vi "to posint fixint.vi"(8 "error in":errorcluster, 11 "bytes":u8[](array[numeric]) format="%b") -> (0 "error out":errorcluster, 2 "fix int":u8, 3 "remaining bytes":u8[](array[numeric]))   [LabVIEW 2020, in "MessagePack.lvlib" / "MessagePack.lvclass"]
uses:
  MessagePack.lvclass
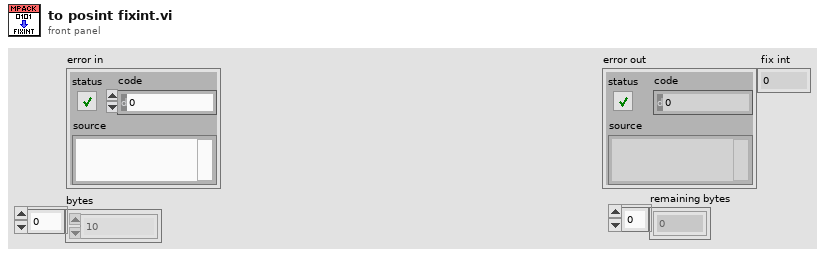
[diagram p1: front panel]
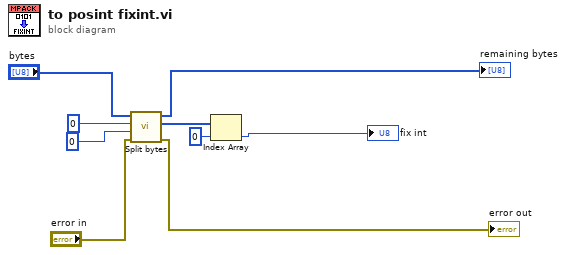
[diagram p0: block diagram]
diagram:
  n1 = call "Split bytes.vi"("error in"="error in", "End index"=0, "Start index"=0, "bytes in"="bytes") -> ("error out"=→"error out":errorcluster, "selected bytes"=w3:u8[], "remaining bytes"=→"remaining bytes":u8[])  [unwired: 4 in, 1 out]
  n2 = Index Array(array=w3, index=0) -> (element=→"fix int":u8)
